vi "Init Response.vi"(8 "error in (no error)":errorcluster, 10 "Result":refnum<class "Acquired Result.lvclass">, 11 "Measure Controller in":refnum<class "Monitor Controller.lvclass">) -> (0 "error out":errorcluster, 3 "Measure Controller out":refnum<class "Monitor Controller.lvclass">)   [LabVIEW 2021, in "Monitor Controller.lvclass"]
uses:
  Monitor Controller.lvclass
  NHMFL_Core/Libraries/Instruments/Results/Acquired Result/Acquired Result.lvclass
  C:/Program Files/National Instruments/LabVIEW 2021/vi.lib/ActorFramework/Actor/Actor.lvclass
  C:/GitHub/LabActor/Worker/Worker Actor/Worker Actor.lvclass
  C:/GitHub/LabActor/Template Module/Template Module.lvclass
  C:/GitHub/LabActor/Controllers/Process Controller/Process Controller.lvclass
  NHMFL_Core/Libraries/Instruments/Instrument Driver/Worker State.ctl
  <vilib>/ActorFramework/Actor/Actor.lvclass/Actor.ctl
  <vilib>/ActorFramework/Message Enqueuer/Message Enqueuer.lvclass/Message Enqueuer.ctl
  Publish-Subscribe/Interfaces/Publisher Messages/Unsubscribe from Topic Msg/Unsubscribe from Topic Msg.lvclass/Unsubscribe from Topic Msg.ctl
  Worker/Worker Actor/Worker Actor.lvclass/Worker Actor.ctl
  Template Module/Template Module.lvclass/Template Module.ctl
  Template Module/Write State.vi
  Template Module/Read Logger.vi
  Template Module/Write Logger.vi
  <vilib>/ActorFramework/Message Enqueuer/Init from Existing Queue.vi
  <vilib>/ActorFramework/Message Enqueuer/Enqueue.vi
  Publish-Subscribe/Interfaces/Publisher Messages/Unsubscribe from Topic Msg/Unsubscribe from Topic Msg.lvclass
  C:/Program Files/National Instruments/LabVIEW 2021/vi.lib/ActorFramework/Message/Message.lvclass
  <vilib>/ActorFramework/Message Priority Queue/Priority Enqueue.vi
  <vilib>/ActorFramework/Message Enqueuer/Message Enqueuer.lvclass
  Loggers/Logger/Logger.lvclass
  <vilib>/ActorFramework/Actor/Actor.lvclass
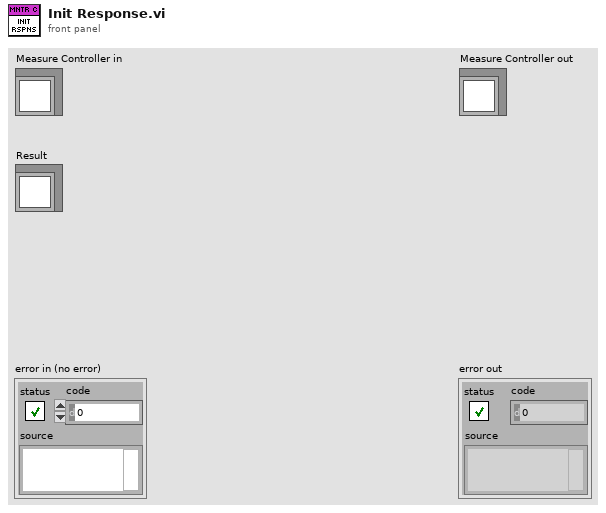
[diagram p1: front panel]
types:
  T1 = typedef "Worker State.ctl" = enum16{"Idle", "Starting", "Working", "Stopping"}
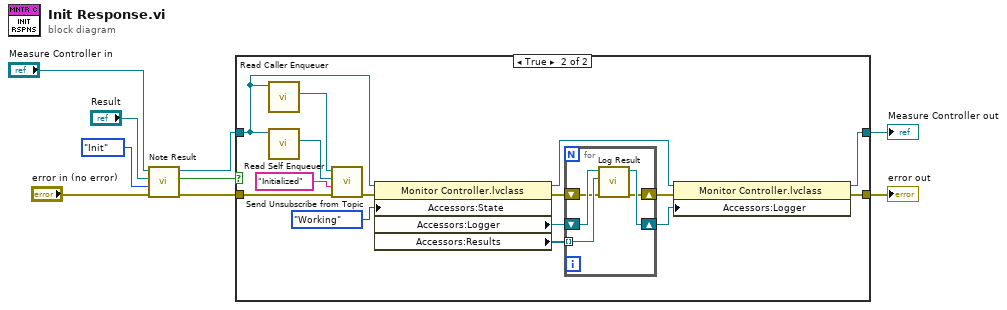
[diagram p0: block diagram]
diagram:
  n1 = call-dynamic "Note Result.vi"("error in (no error)"="error in (no error)", "Stage"=enum16{"Init", "Work"}."Init", "Acquired Result.lvclass"="Result", "Measure Controller in"="Measure Controller in") -> ("error out"=w4:errorcluster, "Result ready"=w5:bool, "Measure Controller out"=w3:refnum<class "Monitor Controller.lvclass">)  [unwired: 5 in]
  n2 = case shown="True" w5 {
    tunnel: w3 -> [w11 w25]
    tunnel: [w11 w16] -> w1
    tunnel: w4 -> [w10 w22]
    tunnel: [w10 w15] -> w2
    frame False {
    }
    frame True {
      n3 = call <vilib>:"Read Caller Enqueuer.vi"("Actor"=w25) -> ("Caller Enqueuer"=w24:refnum<class "Message Enqueuer.lvclass">)  [unwired: 10 in]
      n4 = call <vilib>:"Read Self Enqueuer.vi"("Actor"=w25) -> ("Self Enqueuer"=w23:refnum<class "Message Enqueuer.lvclass">)  [unwired: 10 in]
      n5 = call "Send Unsubscribe from Topic.vi"("error in (no error)"=w22, "Topic"="Initialized", "Subscriber Enq"=w23, "Message Enqueuer"=w24) -> ("error out"=w20:errorcluster)  [unwired: 6 in, 1 out]
      n6 = property class="Monitor Controller.lvclass"(reference=w25, error in=w20, "Accessors:State"=Worker_State."Working" ("State")) -> (reference out=w17:refnum<class "Monitor Controller.lvclass">, error out=w12:errorcluster, "Accessors:Logger"=w18:refnum<class "Logger.lvclass">, "Accessors:Results"=w19:refnum<class "Acquired Result.lvclass">[])
      n7 = for {
        tunnel: w19 -> [w31] mode=indexing
        shift-right: [w29] -> w13
        shift-left: w18 -> [w30]
        shift-right: [w27] -> w14
        shift-left: w12 -> [w28]
        n8 = call-dynamic "Log Result.vi"("error in (no error)"=w28, "Result"=w31, "Logger in"=w30) -> ("error out"=w27:errorcluster, "Logger out"=w29:refnum<class "Logger.lvclass">)  [unwired: 7 in]
      }
      n9 = property class="Monitor Controller.lvclass"(reference=w17, error in=w14, "Accessors:Logger"=w13) -> (reference out=w16:refnum<class "Monitor Controller.lvclass">, error out=w15:errorcluster)
    }
  }
  "error out" <- w2
  "Measure Controller out" <- w1
